vi "Demo v5_QL.vi"() -> ()   [LabVIEW 2013]
panel:
  out "Biggest score":i32
  in  "Reset score":bool
  in  "Reset x":bool
  out "Biggest x":i32
  out "Bird height":i32
  in  "ms to wait":u32=1000
  out "0, 1":i16[](graph)
  out "Out of bound":bool
  out "Hit tube":bool
  out "Unrolled state":i32
  out "Brid x":i32
  out "Iteration":i32
  out "Q":dbl[][](array[numeric])
  in  "Slow":bool=TRUE
  in  "Reset Q":bool
  in  "stop":bool
  out "JUMP?":bool
  out "SCORE":i32
  out "FAIL!":bool
  in  "a":dbl=-0.3
  in  "Jump speed":dbl=3.0
  out "Picture":i32[][](graph)
  # "JUMP"
  # "FALL"
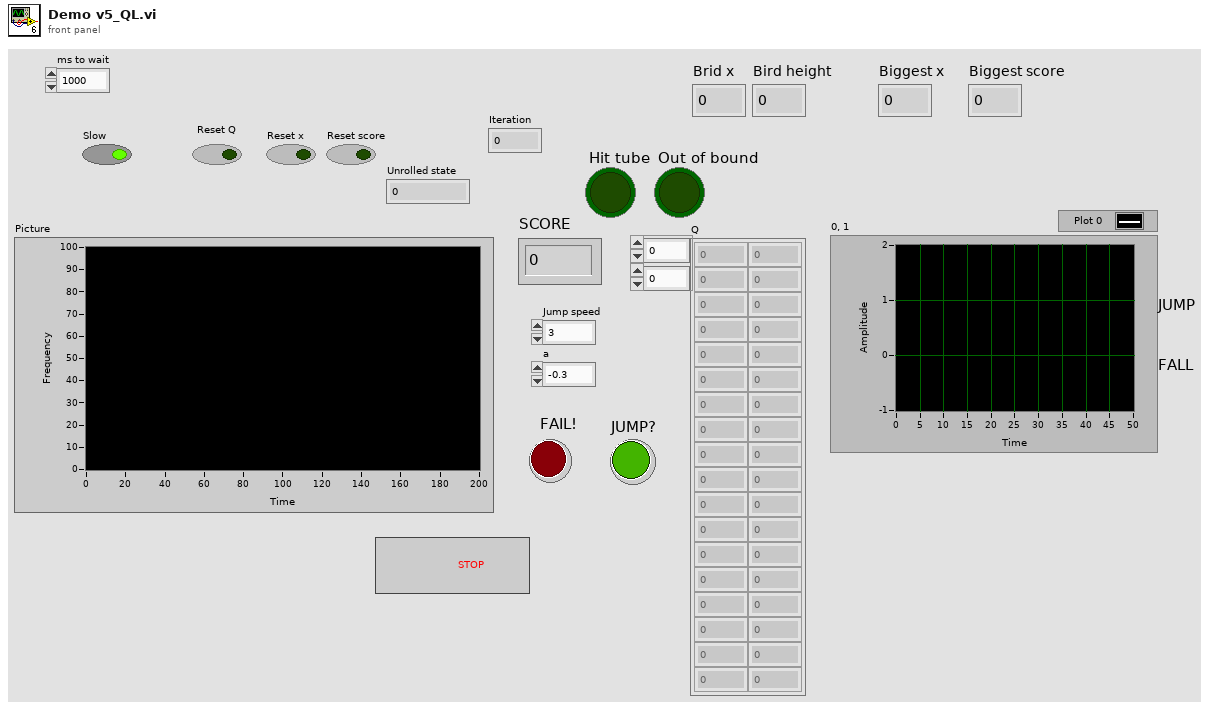
[diagram p1: front panel]
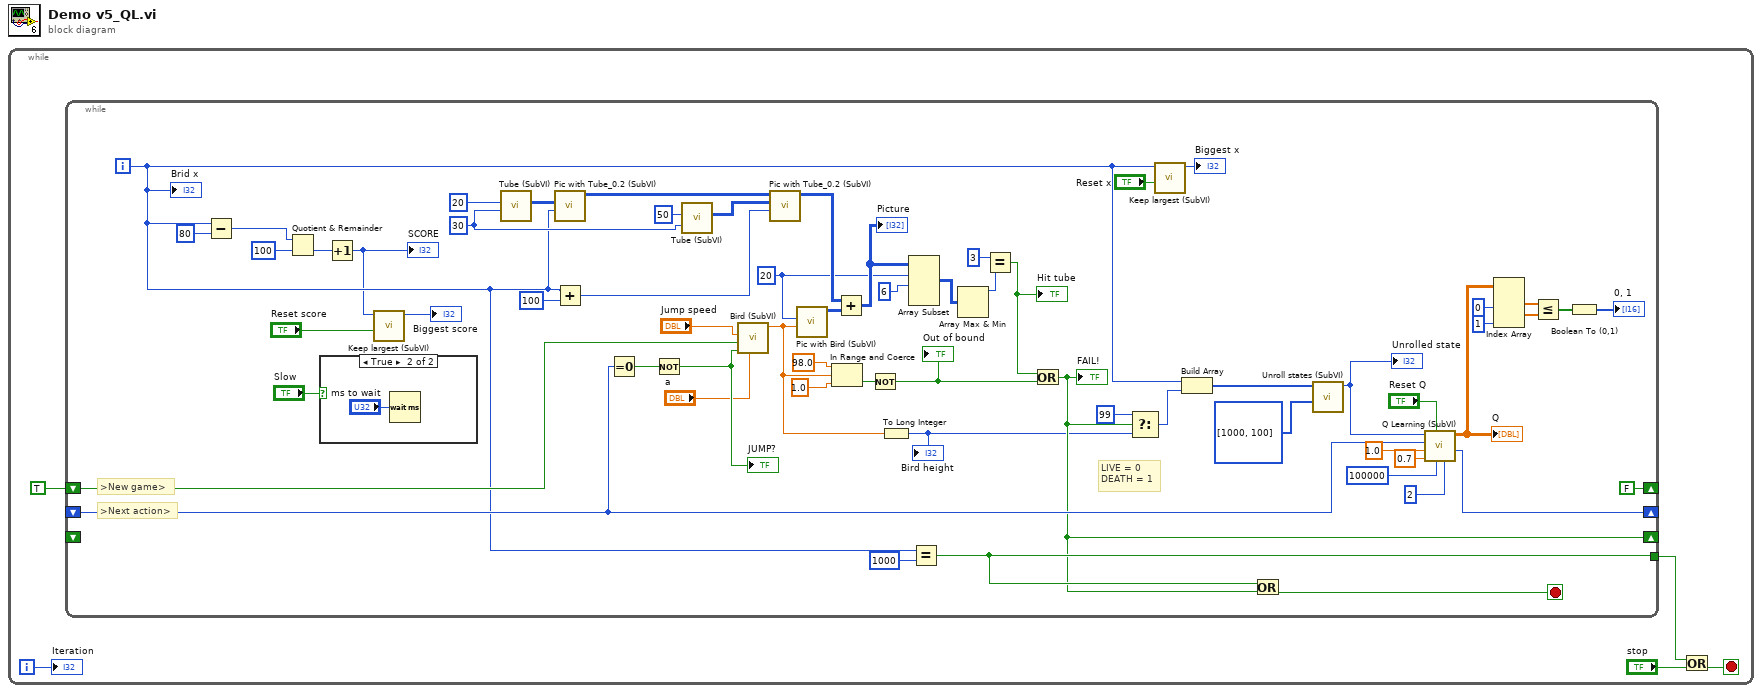
[diagram p0: block diagram]
diagram:
  n1 = while {
    i -> [w4]
    stop <- w3 stop-if-true
    n2 = while {
      shift-right: [w22] -> _
      shift-left: _ -> [_]
      tunnel: [w37] -> w2
      shift-right: [FALSE] -> _
      shift-left: TRUE -> [w27]
      shift-right: [w25] -> _
      shift-left: _ -> [w24]
      i -> [w18]
      stop <- w38 stop-if-true
      w12 = 20 ("X position")
      w64 = 30 ("Gap height (30)")
      # ">New game>"
      # ">Next action>"
      # "LIVE = 0\nDEATH = 1"
      n3 = Subtract(x=w18, y=80) -> (x-y=w56:i32)
      n4 = Quotient & Remainder(x=w56, y=100) -> (floor(x/y)=w8:i32)  [unwired: 1 out]
      n5 = case shown="True" "Slow" {
        frame False {
        }
        frame True {
          n6 = Wait (ms)(milliseconds to wait="ms to wait") -> ()  [unwired: 1 out]
        }
      }
      n7 = Increment(x=w8) -> (x+1=w6:i32)
      "SCORE" <- w6
      n8 = call "Keep largest (SubVI).vi"("Reset"="Reset score", "Input"=w6) -> ("Biggest"=→"Biggest score":i32)  [unwired: 9 in]
      n9 = call "Tube (SubVI).vi"("Gap height (30)"=w64, "Gap low y"=20) -> ("Tube"=w66:i32[][])  [unwired: 9 in]
      n10 = call "Pic with Tube_0.2 (SubVI).vi"("Tube x"=w18, "Tube"=w66) -> ("Picture"=w65:i32[][])  [unwired: 9 in]
      n11 = Add(x=w18, y=100) -> (x+y=w41:i32)
      n12 = Equal To 0?(x=w24) -> (x = 0?=w50:bool)
      n13 = Not(x=w50) -> (.not. x?=w49:bool)
      "JUMP?" <- w49
      n14 = call "Tube (SubVI).vi"("Gap height (30)"=w64, "Gap low y"=50) -> ("Tube"=w29:i32[][])  [unwired: 9 in]
      n15 = call "Bird (SubVI).vi"("a"="a", "Jump"=w49, "Reset"=w27, "Jump speed"="Jump speed") -> ("Position"=w23:dbl)  [unwired: 7 in]
      n16 = call "Pic with Tube_0.2 (SubVI).vi"("Tube x"=w41, "Tube"=w29, "Picture in"=w65) -> ("Picture"=w44:i32[][])  [unwired: 8 in]
      n17 = call "Pic with Bird (SubVI).vi"("Bird Position"=w23, "X position"=w12) -> ("Picture"=w68:i32[][])  [unwired: 9 in]
      n18 = In Range and Coerce(upper limit=98.0, x=w23, lower limit=1.0) -> (In Range?=w61:bool)  [unwired: 1 out]
      n19 = Add(x=w44, y=w68) -> (x+y=w13:i32[][])
      "Picture" <- w13
      n20 = Not(x=w61) -> (.not. x?=w59:bool)
      "Out of bound" <- w59
      n21 = To Long Integer(number=w23) -> (32bit integer=w21:i32)
      "Bird height" <- w21
      n22 = Array Subset(array=w13, index (row)=w12, length (row)=6 ("length")) -> (w10:i32[][])  [unwired: 2 in]
      n23 = Equal?(x=w18, y=1000) -> (x = y?=w37:bool)
      n24 = Array Max & Min(array=w10) -> (max value=w9:i32)  [unwired: 3 out]
      n25 = Equal?(x=3 ("y"), y=w9) -> (x = y?=w45:bool)
      "Hit tube" <- w45
      n26 = Or(x=w45, y=w59) -> (x .or. y?=w22:bool)
      "FAIL!" <- w22
      n27 = Select(t=99, s=w22, f=w21) -> (s? t:f=w20:i32)
      n28 = call "Keep largest (SubVI).vi"("Reset"="Reset x", "Input"=w18) -> ("Biggest"=→"Biggest x":i32)  [unwired: 9 in]
      n29 = Build Array(w18, w20) -> (w51:i32[])
      n30 = Or(x=w37, y=w22) -> (x .or. y?=w38:bool)
      n31 = call "Unroll states (SubVI).vi"("# each state"=i32[] [1000, 100], "State array"=w51) -> ("Unrolled state"=w16:i32)  [unwired: 9 in]
      "Unrolled state" <- w16
      n32 = call "Q Learning (SubVI).vi"("# action"=2, "# state"=100000, "Reset"="Reset Q", "alpha"=0.7, "Gamma"=1.0, "Action"=w24, "State"=w16) -> ("Next Action"=w25:i32, "Q"=w36:dbl[][])  [unwired: 3 in]
      "Q" <- w36
      n33 = Index Array(array=w36, index (col) #1=0 ("disabled index (col)"), index (col) #2=1 ("index (col)")) -> (element #1=w33:dbl[], element #2=w32:dbl[])  [unwired: 2 in]
      n34 = Less Or Equal?(x=w33, y=w32) -> (x <= y?=w31:bool[])
      n35 = Boolean To (0,1)(Boolean=w31) -> (0, 1=→"0, 1":i16[])
      "Brid x" <- w18
    }
    n36 = Or(x=w2, y="stop") -> (x .or. y?=w3:bool)
    "Iteration" <- w4
  }
